vi "Write connection settings.vi"(8 "error in (no error)":errorcluster, 10 "connection settings":T1={"Com"="", "baud rate (9600)"=38400} {"baud rate (9600)" items=["75"=75, "110"=110, "134"=134, "150"=150, "300"=300, "600"=600, "1200"=1200, "1800"=1800, "2400"=2400, "4800"=4800, "7200"=7200, "9600"=9600, "14400"=14400, "19200"=19200, "28800"=28800, "38400"=38400, "56000"=56000, "57600"=57600, "115200"=115200, "128000"=128000, "230400"=230400]}, 11 "VD-LV-LiteVNA in":refnum<class "VD-LV-LiteVNA.lvclass">) -> (0 "error out":errorcluster, 3 "VD-LV-LiteVNA out":refnum<class "VD-LV-LiteVNA.lvclass">)   [LabVIEW 2020, in "VD-LV-LiteVNA.lvclass"]
uses:
  VD-LV-LiteVNA.lvclass
  VD-connection_settings.ctl
  hardware-protocol/serial/HP-S-baudrate.ctl
  VD-LV-LiteVNA.lvclass/VD-LV-LiteVNA.ctl
  hardware-protocol/serial/HP-S-Serial.lvclass
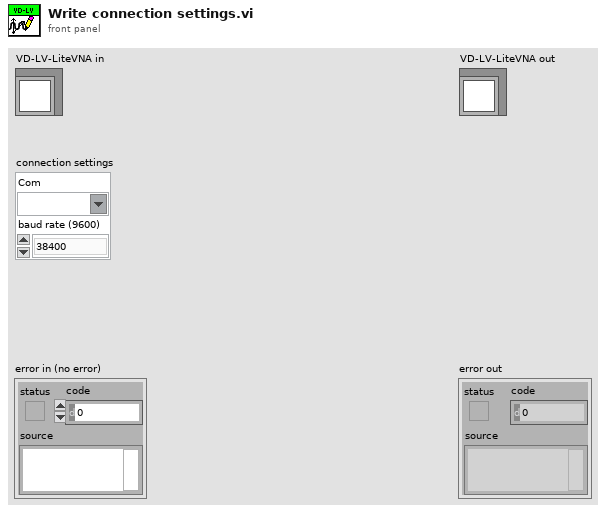
[diagram p1: front panel]
types:
  T1 = typedef "VD-LV-LiteVNA.lvclass/VD-connection_settings.ctl" = cluster{"Com":refnum<visa-resource-name>, "baud rate (9600)":T2}
  T2 = typedef "HP-S-Serial.lvclass/HP-S-baudrate.ctl" = u32
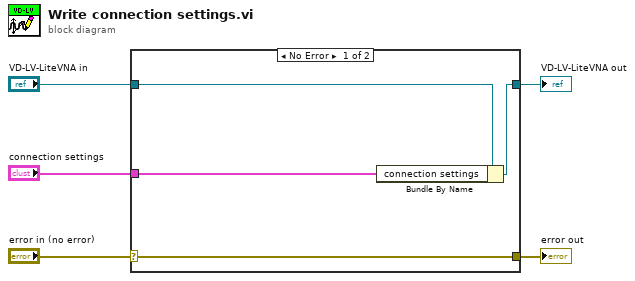
[diagram p0: block diagram]
diagram:
  n1 = case shown="No Error" "error in (no error)" {
    selector: "error in (no error)" -> [w9 w10]
    tunnel: [w9 w10] -> w4
    tunnel: [w7 w11] -> w2
    tunnel: "VD-LV-LiteVNA in" -> [w8 w11]
    tunnel: "connection settings" -> [w6 _]
    frame No Error {
      n2 = Bundle By Name(cluster=w8, "connection settings"=w6) -> (w7:refnum<class "VD-LV-LiteVNA.lvclass">)
    }
    frame Error {
    }
  }
  "error out" <- w4
  "VD-LV-LiteVNA out" <- w2
